vi "subGeneratePackets.vi"(0 "调制方式":enum32{"PSK", "FSK"}(tab), 1 "Tx IQ Sampling\nRate [s/sec]":dbl, 3 "Samples per Symbol":i32, 4 "Pulse Shaping Filter Parameters":T4, 5 "Packet Repeat":i32, 7 "PN sequence order\nfor Sync Bits":i32, 8 "FSK system parameters":T1 {"symbol map" format="%.2f"}, 9 "Packet Parameters":T2, 10 "Packet Pad \n[samples]":i32, 16 "PSK system parameters":T3, 27 "Message Text":string) -> (20 "Number of Packets":i32, 21 "Packets":cluster{"t0":dbl, "dt":dbl, "Y":cdb[]}[](array[cluster]), 25 "Symbol Rate":dbl)   [LabVIEW 2015]
uses:
  <vilib>/addons/Modulation/Digital/Support/Controls/FSK System Parameters.ctl
  <vilib>/addons/Modulation/niDMT.lvlib
panel:
  in  "调制方式选择":enum32{"PSK", "FSK"}(tab)
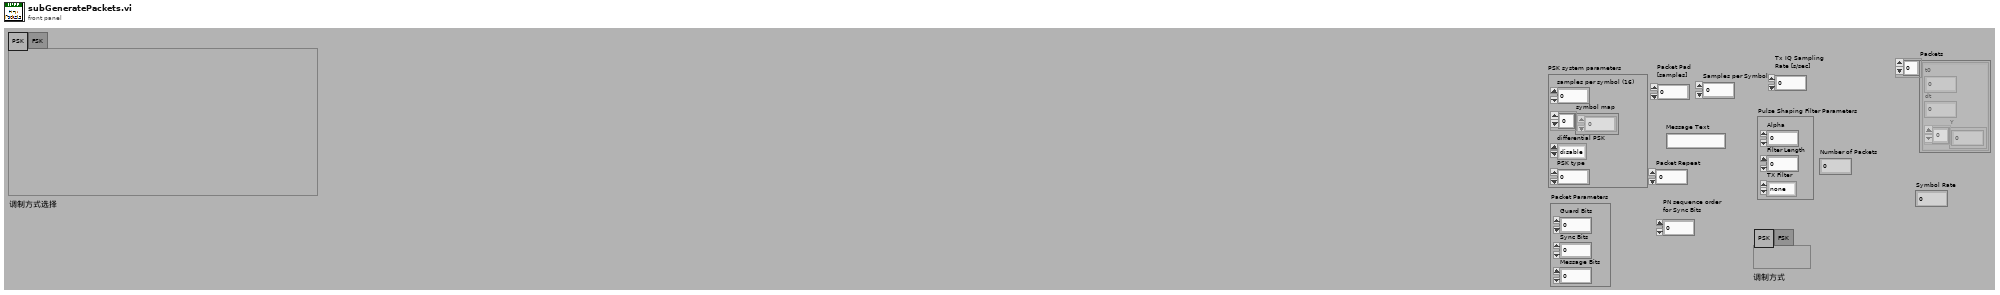
[diagram p1: front panel]
types:
  T1 = typedef "niDMT.lvlib/FSK System Parameters.ctl" = cluster{"samples per symbol (16)":i32, "symbol map":dbl[], "symbol phase continuity":enum16{"continuous", "discontinuous"}}
  T2 = cluster{"Guard Bits ":i32, "Sync Bits":i32, "Message Bits":i32}
  T3 = cluster{"samples per symbol (16)":i32, "symbol map":cdb[], "differential PSK":enum16{"disable", "enable"}, "PSK type":u16}
  T4 = cluster{"Alpha":dbl, "Filter Length":i32, "TX Filter":enum16{"none", "Raised Cosine", "Root Raised Cos", "Gaussian"}}
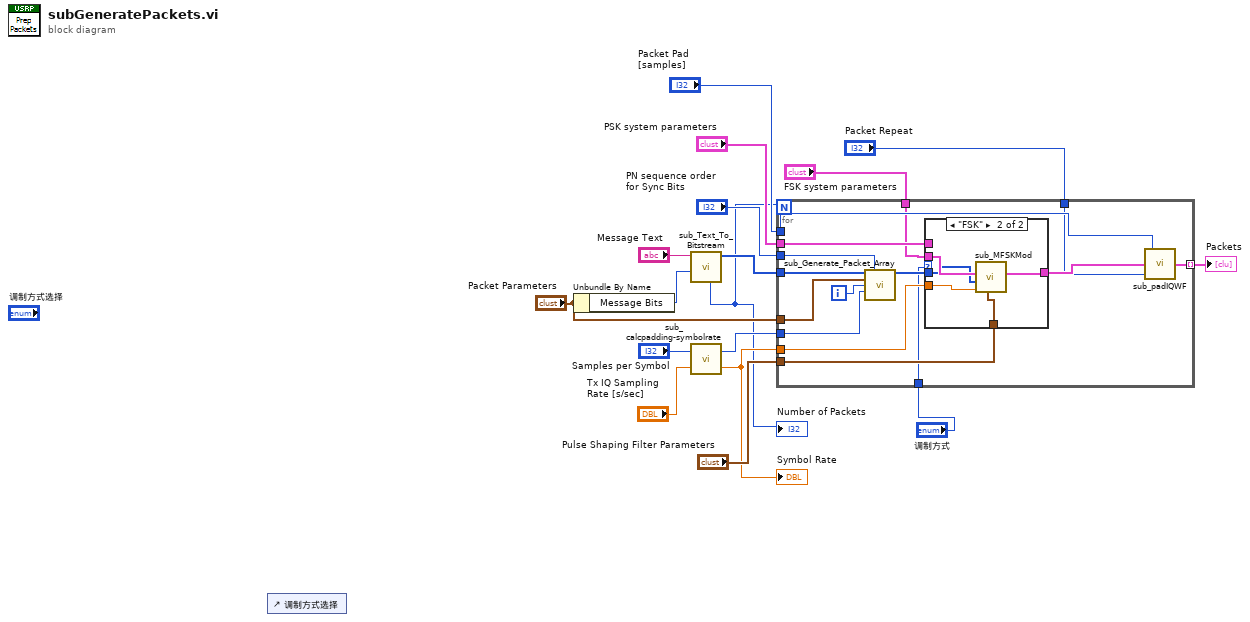
[diagram p0: block diagram]
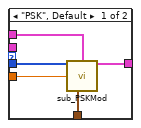
[diagram p2: hidden frame]
diagram:
  n1 = control-ref of="调制方式选择"() -> ()  [unwired: 1 out]
  n2 = Unbundle By Name("Packet Parameters") -> ("Message Bits"=w9:i32)
  n3 = call "sub_Text_To_Bitstream.vi"("Packet\nMessage Length (bits)"=w9, "text"="Message Text") -> ("message bitstream"=w13:i8[], "Number of Packets"=w4:i32)  [unwired: 7 in, 1 out]
  "Number of Packets" <- w4
  n4 = call "sub_calcpadding-symbolrate.vi"("Tx IQ Sampling\nRate [s/sec]"="Tx IQ Sampling\nRate [s/sec]", "Samples per Symbol"="Samples per Symbol") -> ("Symbol Rate"=w6:dbl, "Padding Bits"=w8:i32)
  "Symbol Rate" <- w6
  n5 = for {
    N: w4 -> [_]
    tunnel: "Packet Parameters" -> [w21]
    tunnel: [w26] -> w11 mode=indexing
    tunnel: w13 -> [w23]
    tunnel: "PN sequence order\nfor Sync Bits" -> [w31]
    tunnel: w8 -> [w22]
    tunnel: "PSK system parameters" -> [w29]
    tunnel: w6 -> [w28]
    tunnel: "Pulse Shaping Filter Parameters" -> [w27]
    tunnel: "Packet Pad \n[samples]" -> [w24]
    tunnel: "Packet Repeat" -> [w20]
    tunnel: "调制方式" -> [w19]
    tunnel: "FSK system parameters" -> [w18]
    i -> [w32]
    n6 = call "sub_Generate_Packet_Array.vi"("user  bitstream"=w23, "PN sequence order\nfor Sync"=w31, "Packet Parameters"=w21, "Packet Number"=w32, "Cyclic Padding Bits"=w22) -> ("Output Packet"=w30:i8[])  [unwired: 10 in]
    n7 = case shown="\"FSK\"" w19 {
      tunnel: w30 -> [w37 w41]
      tunnel: w29 -> [w36 _]
      tunnel: w28 -> [w35 w39]
      tunnel: w27 -> [w34 w38]
      tunnel: [w33 w40] -> w25
      tunnel: w18 -> [_ w42]
      frame "PSK", Default {
        n8 = call "sub_PSKMod.vi"("Packet to Transmit"=w37, "PSK system parameters"=w36, "Symbol Rate, Hz"=w35, "filter parameters"=w34) -> ("output complex waveform"=w33:cluster{"t0":dbl, "dt":dbl, "Y":cdb[]})  [unwired: 10 in, 1 out]
      }
      frame "FSK" {
        n9 = call "sub_MFSKMod.vi"("filter parameters"=w38, "Symbol Rate, Hz"=w39, "Packet to Transmit"=w41, "FSK system parameters"=w42) -> ("output complex waveform"=w40:cluster{"t0":dbl, "dt":dbl, "Y":cdb[]})  [unwired: 7 in]
      }
    }
    n10 = call "sub_padIQWF.vi"("Repeat"=w20, "input complex waveform"=w25, "Packet Pad \n[samples]"=w24) -> ("output complex waveform"=w26:cluster{"t0":dbl, "dt":dbl, "Y":cdb[]})
  }
  "Packets" <- w11
